vi "Write Log File Path.vi"(8 "error in (no error)":errorcluster, 10 "Log File Path":path, 11 "Abstract Log Init Parameters in":refnum<class "Abstract Log Init Parameters.lvclass">) -> (0 "error out":errorcluster, 3 "Abstract Log Init Parameters out":refnum<class "Abstract Log Init Parameters.lvclass">)   [LabVIEW 2017, in "Messaging.lvlib" / "Abstract Log Init Parameters.lvclass"]
uses:
  Abstract Log Init Parameters.lvclass
  Abstract Log Init Parameters.lvclass/Abstract Log Init Parameters.ctl
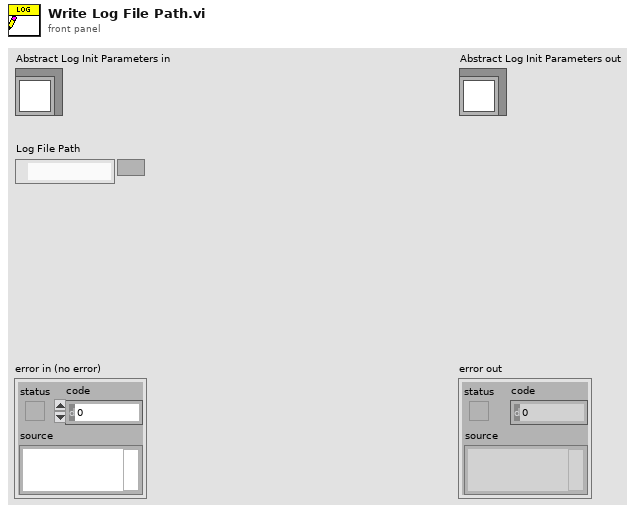
[diagram p1: front panel]
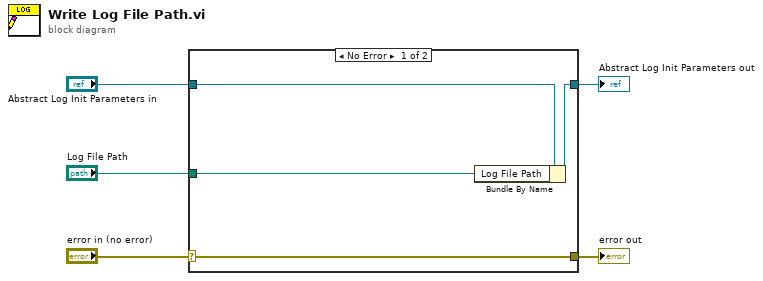
[diagram p0: block diagram]
diagram:
  n1 = case shown="No Error" "error in (no error)" {
    selector: "error in (no error)" -> [w9 w10]
    tunnel: [w9 w10] -> w4
    tunnel: [w7 w11] -> w2
    tunnel: "Abstract Log Init Parameters in" -> [w8 w11]
    tunnel: "Log File Path" -> [w6 _]
    frame No Error {
      n2 = Bundle By Name(cluster=w8, "Log File Path"=w6) -> (w7:refnum<class "Abstract Log Init Parameters.lvclass">)
    }
    frame Error {
    }
  }
  "error out" <- w4
  "Abstract Log Init Parameters out" <- w2
